vi "Wait Until Cancelled or Complete.vi"(6 "done channel":T2, 8 "error in (no error)":errorcluster, 9 "ms polling interval":i32=100, 11 "measure call context in":refnum<class "Measure Call Context.lvclass">) -> (0 "error out":errorcluster, 3 "measure call context out":refnum<class "Measure Call Context.lvclass">, 4 "stop channel":T1)   [LabVIEW 2024, in "Dynamic Signal Acquisition (Interactive).lvlib"]
doc: "Monitor for cancellation and abort the measurement if a cancellation request is received before the measurement completes normally."
uses:
  Dynamic Signal Acquisition (Interactive).lvlib
  <vilib>/Plug-In SDKs/Measurements/Measure Call Context/Measure Call Context.lvclass
  <extravilib>/ChannelInstances/Event Messenger-bool/))Channel.ctl
  <extravilib>/ChannelInstances/Tag-bool/Read.vi
  <extravilib>/ChannelInstances/Tag-bool/Write.vi
  <extravilib>/ChannelInstances/Tag-bool/Read With Abort.vi
  <extravilib>/ChannelInstances/Tag-bool/Write With Abort.vi
  <extravilib>/ChannelInstances/Event Messenger-bool/))Channel.vi
  <extravilib>/ChannelInstances/Tag-bool/Instantiate.vi
  <extravilib>/ChannelInstances/Tag-bool/EndpointRead.vi
  <extravilib>/ChannelInstances/Tag-bool/Endpoint.vi
  <extravilib>/ChannelInstances/Event Messenger-bool.lvlib
  <extravilib>/ChannelInstances/Tag-bool/))Channel.ctl
  <extravilib>/ChannelInstances/Tag-bool.lvlib
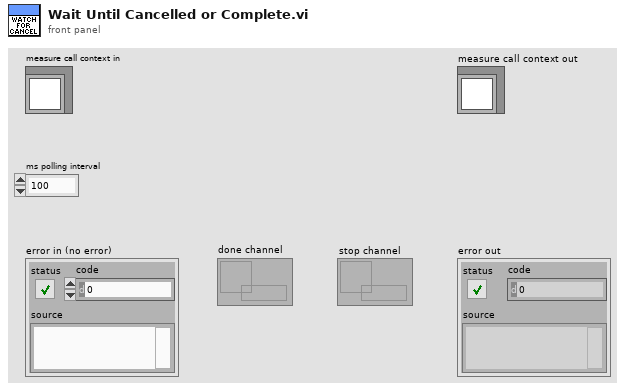
[diagram p1: front panel]
types:
  T1 = typedef "Tag-bool.lvlib/))Channel.ctl" = refnum<queue>
  T2 = typedef "Event Messenger-bool.lvlib/))Channel.ctl" = refnum<queue>
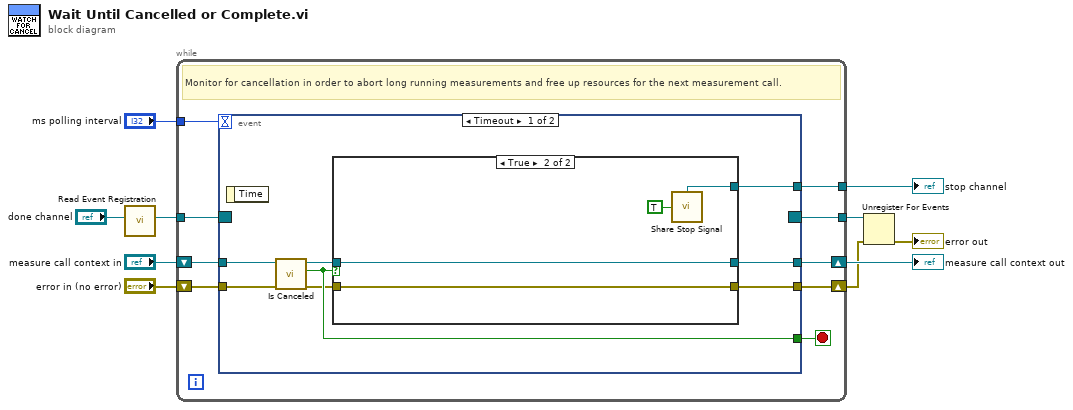
[diagram p0: block diagram]
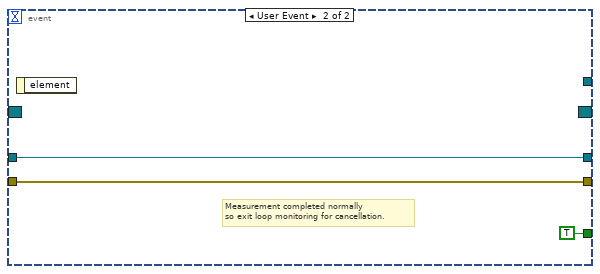
[diagram p3: hidden frame]
diagram:
  n1 = call <extravilib>:"Read Event Registration.vi"("channel"="done channel") -> ("event registration refnum"=w6:refnum<event-registration>)  [unwired: 10 in]
  n2 = while {
    shift-right: [w18] -> w10
    shift-left: "measure call context in" -> [w19]
    shift-right: [w15] -> w3
    shift-left: "error in (no error)" -> [w16]
    tunnel: w6 -> [w14]
    tunnel: "ms polling interval" -> [w13]
    tunnel: [w12] -> w4
    tunnel: "stop channel" -> [w11]
    stop <- w17 stop-if-true
    # "Monitor for cancellation in order to abort long running measurements and free up resources for the next measurement call."
    n3 = event shown="[0] Timeout" {
      selector: w14 -> [_ _]
      dyn-events: [_ _] -> w12
      timeout: w13 -> [_ _]
      tunnel: w19 -> [w27 w34]
      tunnel: [w26 w34] -> w18
      tunnel: [w25 TRUE ("is canceled?")] -> w17
      tunnel: w16 -> [w24 w35]
      tunnel: [w23 w35] -> w15
      tunnel: w11 -> [w20 _]
      event Timeout {
        n4 = event-data() -> ()  [unwired: 1 in, 1 out]
        n5 = call <vilib>:"Is Canceled.vi"("error in"=w24, "measure call context in"=w27) -> ("error out"=w22:errorcluster, "is canceled?"=w25:bool, "measure call context out"=w21:refnum<class "Measure Call Context.lvclass">)  [unwired: 7 in]
        n6 = case shown="True" w25 {
          tunnel: w22 -> [w29 w32]
          tunnel: w21 -> [w28 w33]
          tunnel: [w29 w32] -> w23
          tunnel: [w28 w33] -> w26
          tunnel: w20 -> [_ w31]
          frame False {
          }
          frame True {
            n7 = call <vilib>:"Share Stop Signal.vi"("set stop (F)"=TRUE, "channel"=w31) -> ()  [unwired: 1 out]
          }
        }
      }
      event User Event {
        # "Measurement completed normally\nso exit loop monitoring for cancellation."
        n8 = event-data() -> ()  [unwired: 1 in, 1 out]
      }
    }
  }
  "measure call context out" <- w10
  n9 = Unregister For Events(event registration refnum=w4, error in=w3) -> (error out=→"error out":errorcluster)
